vi "Call Instruments.vi"(8 "error in (no error)":errorcluster, 10 "Instrument?":string, 11 "Diagnostic in":refnum<class "Diagnostic.lvclass">) -> (0 "error out":errorcluster, 3 "Diagnostic out":refnum<class "Diagnostic.lvclass">)   [LabVIEW 2023, in "GUI.lvlib" / "Diagnostic.lvlib" / "Diagnostic.lvclass"]
uses:
  Diagnostic.lvclass
  Instruments UI/PowerSupply/PPS User Interface.vi
  Instruments UI/Digital Input/Digital Input User Interface.vi
  Instruments UI/Digital Output/Digital Output User Interface.vi
  Instruments UI/Analog Input/Analog Input User Interface.vi
  Instruments UI/Analog Output/Analog Output User Interface.vi
  Instruments UI/Waveform Generation/Waveform Generation User Interface.vi
  Instruments UI/PWM Input/PWM Input User Interface.vi
  Instruments UI/PWM Output/PWM Output User Interface.vi
  Instruments UI/Relay Output/Realy Output User Interface.vi
  Instruments UI/CAN/VAL SW Testing/Validate VAL SW.vi
  Database Configuration/DAQ/Database Configuration.vi
  Instruments UI/Temparature Controller/Temperature User Interface.vi
  Diagnostic.lvlib
  Instruments UI/CAN/VAL SW Testing/VAL_SW_Testing.lvlib
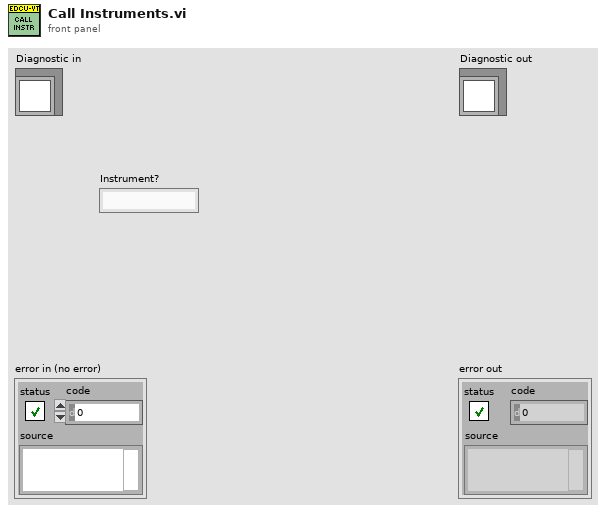
[diagram p1: front panel]
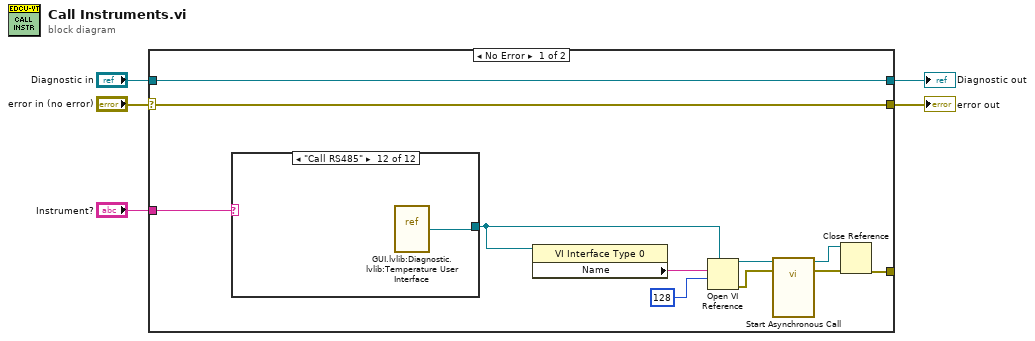
[diagram p0: block diagram]
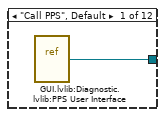
[diagram p2: hidden frame]
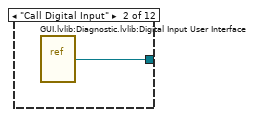
[diagram p3: hidden frame]
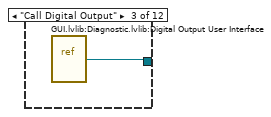
[diagram p4: hidden frame]
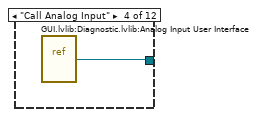
[diagram p5: hidden frame]
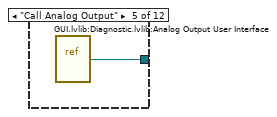
[diagram p6: hidden frame]
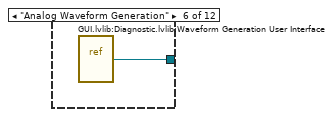
[diagram p7: hidden frame]
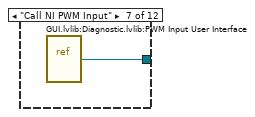
[diagram p8: hidden frame]
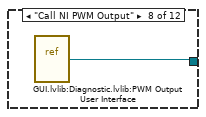
[diagram p9: hidden frame]
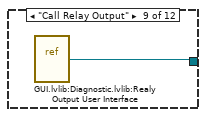
[diagram p10: hidden frame]
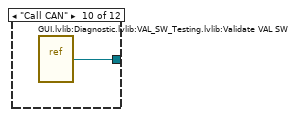
[diagram p11: hidden frame]
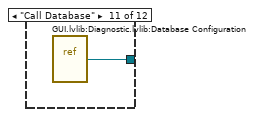
[diagram p12: hidden frame]
diagram:
  n1 = case shown="No Error" "error in (no error)" {
    selector: "error in (no error)" -> [w15 w30]
    tunnel: [w15 w30] -> w4
    tunnel: [w16 w29] -> w2
    tunnel: "Diagnostic in" -> [w16 w29]
    tunnel: "Instrument?" -> [w8 _]
    tunnel: [w12 _] -> _
    frame No Error {
      n2 = case shown="\"Call RS485\"" w8 {
        tunnel: [w17 w18 w19 w20 w21 w22 w23 w24 w25 w26 w27 w28] -> w7
        frame "Call PPS", Default {
          n3 = vi-ref "GUI.lvlib:Diagnostic.lvlib:PPS User Interface.vi"() -> (w17:refnum<vi>)
        }
        frame "Call Digital Input" {
          n4 = vi-ref "GUI.lvlib:Diagnostic.lvlib:Digital Input User Interface.vi"() -> (w18:refnum<vi>)
        }
        frame "Call Digital Output" {
          n5 = vi-ref "GUI.lvlib:Diagnostic.lvlib:Digital Output User Interface.vi"() -> (w19:refnum<vi>)
        }
        frame "Call Analog Input" {
          n6 = vi-ref "GUI.lvlib:Diagnostic.lvlib:Analog Input User Interface.vi"() -> (w20:refnum<vi>)
        }
        frame "Call Analog Output" {
          n7 = vi-ref "GUI.lvlib:Diagnostic.lvlib:Analog Output User Interface.vi"() -> (w21:refnum<vi>)
        }
        frame "Analog Waveform Generation" {
          n8 = vi-ref "GUI.lvlib:Diagnostic.lvlib:Waveform Generation User Interface.vi"() -> (w22:refnum<vi>)
        }
        frame "Call NI PWM Input" {
          n9 = vi-ref "GUI.lvlib:Diagnostic.lvlib:PWM Input User Interface.vi"() -> (w23:refnum<vi>)
        }
        frame "Call NI PWM Output" {
          n10 = vi-ref "GUI.lvlib:Diagnostic.lvlib:PWM Output User Interface.vi"() -> (w24:refnum<vi>)
        }
        frame "Call Relay Output" {
          n11 = vi-ref "GUI.lvlib:Diagnostic.lvlib:Realy Output User Interface.vi"() -> (w25:refnum<vi>)
        }
        frame "Call CAN" {
          n12 = vi-ref "GUI.lvlib:Diagnostic.lvlib:VAL_SW_Testing.lvlib:Validate VAL SW.vi"() -> (w26:refnum<vi>)
        }
        frame "Call Database" {
          n13 = vi-ref "GUI.lvlib:Diagnostic.lvlib:Database Configuration.vi"() -> (w27:refnum<vi>)
        }
        frame "Call RS485" {
          n14 = vi-ref "GUI.lvlib:Diagnostic.lvlib:Temperature User Interface.vi"() -> (w28:refnum<vi>)
        }
      }
      n15 = property class="VI Interface Type 0"(reference=w7) -> ("Name"=w14:string)  [unwired: 1 in, 2 out]
      n16 = Open VI Reference(type specifier VI Refnum (for type only)=w7, vi path=w14, options=128) -> (vi reference=w6:refnum<vi>, error out=w11:errorcluster)  [unwired: 3 in]
      n17 = call-by-ref "Start Asynchronous Call"(reference=w6, error in=w11) -> (reference out=w9:refnum<vi>, error out=w10:errorcluster)  [unwired: 12 in]
      n18 = Close Reference(reference=w9, error in (no error)=w10) -> (error out=w12:errorcluster)
    }
    frame Error {
    }
  }
  "error out" <- w4
  "Diagnostic out" <- w2
